vi "Get Server DLL Path.vi"() -> (0 "Server dll path":path)   [LabVIEW 2019, in "OCV.lvlib" / "gprc-lvsupport.lvlib"]
uses:
  gprc-lvsupport.lvlib
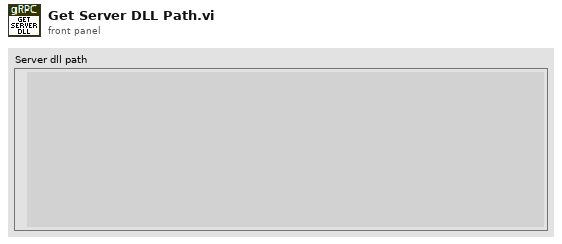
[diagram p1: front panel]
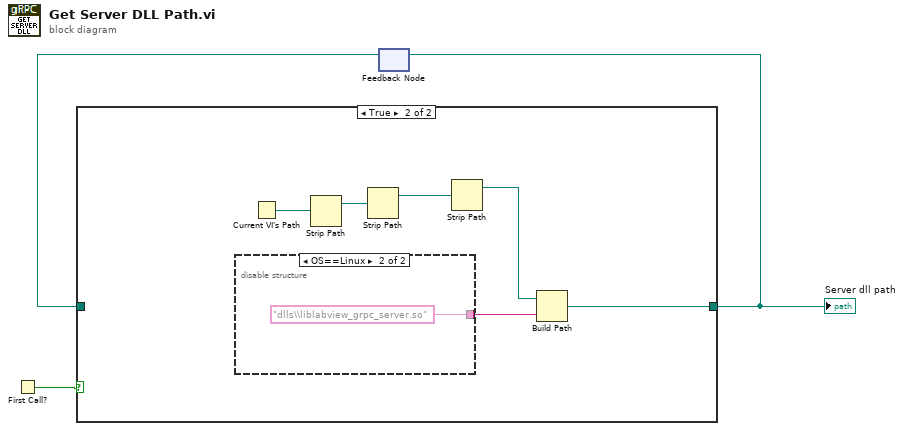
[diagram p0: block diagram]
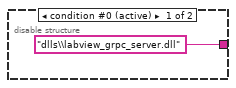
[diagram p3: hidden frame]
diagram:
  n1 = First Call?() -> (First Call?: T/F=w3:bool)
  n2 = feedback #1() -> (w1:path)  [unwired: 1 in]
  n3 = case shown="True" w3 {
    tunnel: [w4 w7] -> w2
    tunnel: w1 -> [w4 _]
    frame False {
    }
    frame True {
      n4 = disable-structure shown="OS==Linux" {
        disable-tunnel: ["dlls\\labview_grpc_server.dll" ("name or relative path") "dlls\\liblabview_grpc_server.so" ("name or relative path")] -> w8
        frame condition #0 (active) {
        }
        frame condition #1 {
        }
      }
      n5 = Current VI's Path() -> (path=w9:path)
      n6 = Strip Path(path=w9) -> (stripped path=w10:path)  [unwired: 1 out]
      n7 = Strip Path(path=w10) -> (stripped path=w6:path)  [unwired: 1 out]
      n8 = Strip Path(path=w6) -> (stripped path=w5:path)  [unwired: 1 out]
      n9 = Build Path(base path=w5, name or relative path=w8) -> (appended path=w7:path)
    }
  }
  "Server dll path" <- w2
  n10 = feedback-in #1(w2) -> ()
